vi "Part 3.vi"() -> ()   [LabVIEW 2016]
panel:
  in  "stop":bool
  out "4":bool
  out "3":bool
  out "2":bool
  out "1":bool
  in  "Press":bool
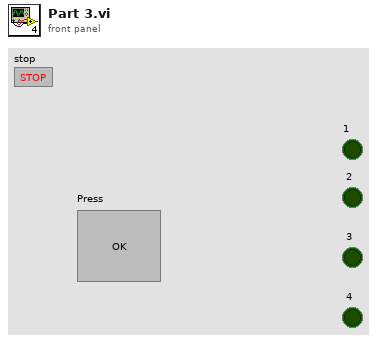
[diagram p1: front panel]
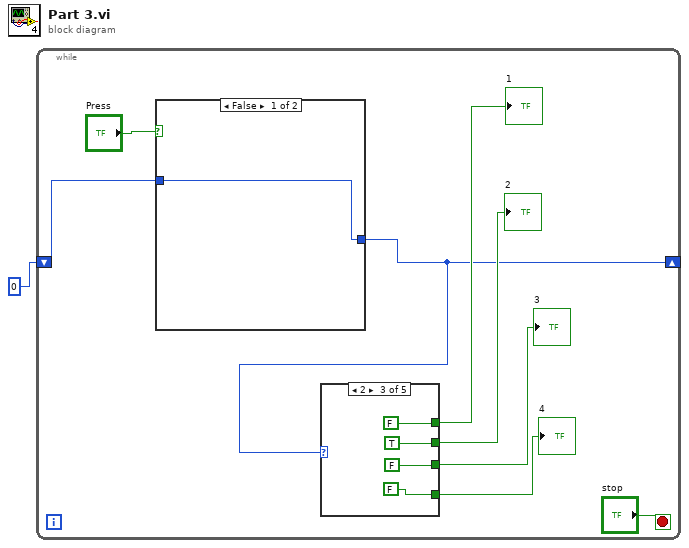
[diagram p0: block diagram]
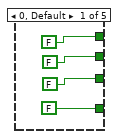
[diagram p2: hidden frame]
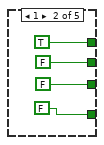
[diagram p3: hidden frame]
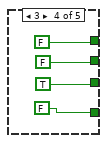
[diagram p4: hidden frame]
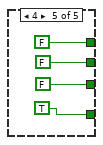
[diagram p5: hidden frame]
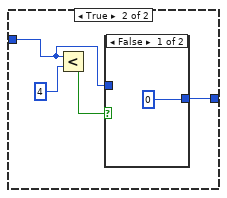
[diagram p6: hidden frame]
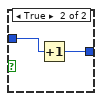
[diagram p7: hidden frame]
diagram:
  n1 = while {
    shift-right: [w3] -> _
    shift-left: 0 -> [w7]
    stop <- "stop" stop-if-true
    n2 = case shown="False" "Press" {
      tunnel: w7 -> [w30 w31]
      tunnel: [w30 w32] -> w3
      frame False {
      }
      frame True {
        n3 = Less?(x=w31, y=4) -> (x < y?=w33:bool)
        n4 = case shown="False" w33 {
          tunnel: [0 w37] -> w32
          tunnel: w31 -> [_ w36]
          frame False {
          }
          frame True {
            n5 = Increment(x=w36) -> (x+1=w37:i32)
          }
        }
      }
    }
    n6 = case shown="2" w3 {
      tunnel: [FALSE TRUE FALSE FALSE FALSE] -> w6
      tunnel: [FALSE FALSE TRUE FALSE FALSE] -> w5
      tunnel: [FALSE FALSE FALSE TRUE FALSE] -> w4
      tunnel: [FALSE FALSE FALSE FALSE TRUE] -> w2
      frame 0, Default {
      }
      frame 1 {
      }
      frame 2 {
      }
      frame 3 {
      }
      frame 4 {
      }
    }
    "1" <- w6
    "2" <- w5
    "3" <- w4
    "4" <- w2
  }
